vi "buildTable.vi"(10 "Locations":dbl[](array[numeric]), 11 "Amplitudes":dbl[](array[numeric])) -> (3 "Table":string[][](array[string]))   [LabVIEW 2014]
doc: "Random Laser Project\nAndré Romero - 2020\nandretec@ifsc.usp.br\n\nBuild data table"
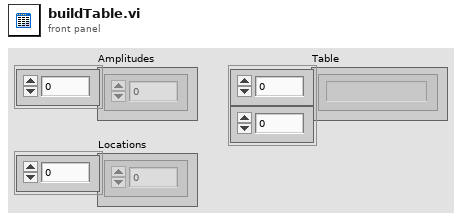
[diagram p1: front panel]
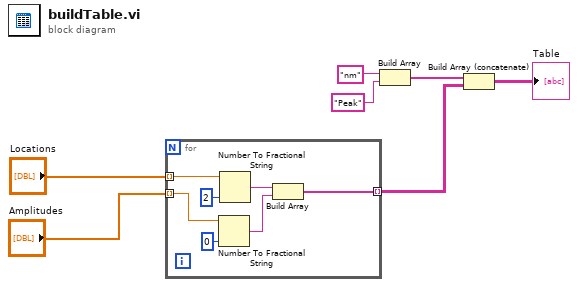
[diagram p0: block diagram]
diagram:
  n1 = for {
    tunnel: "Locations" -> [w14] mode=indexing
    tunnel: "Amplitudes" -> [w13] mode=indexing
    tunnel: [w10] -> w6 mode=indexing
    n2 = Number To Fractional String(number=w13, precision (6)=i16 0) -> (F-format string=w11:string)  [unwired: 2 in]
    n3 = Number To Fractional String(number=w14, precision (6)=i16 2) -> (F-format string=w12:string)  [unwired: 2 in]
    n4 = Build Array(w12, w11) -> (w10:string[])
  }
  n5 = Build Array("nm", "Peak") -> (w5:string[])
  n6 = Build Array (concatenate)(w5, w6) -> (→"Table":string[][])
